vi "apply settings.vi"(8 "error in (no error)":errorcluster, 9 "selectors":T1, 10 "settings":string, 11 "refnum":refnum<vi>) -> (0 "error out":errorcluster)   [LabVIEW 2024, in "controls manager.lvlib"]
uses:
  controls manager.lvlib
  selectors.ctl
  <vilib>/Utility/error.llb/Trim Whitespace One-Sided.vi
  <vilib>/Utility/error.llb/Error Cluster From Error Code.vi
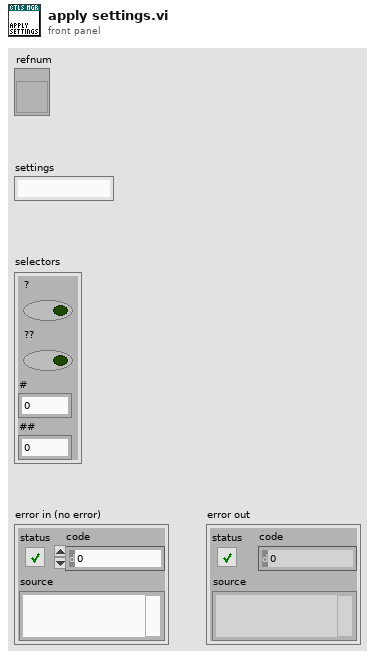
[diagram p1: front panel]
types:
  T1 = typedef "controls manager.lvlib/selectors.ctl" = cluster{"?":bool, "??":bool, "#":u16, "##":u16}
  T2 = enum8{"Enabled", "Disabled", "Disabled and Grayed Out"}
  T3 = typedef "controls manager.lvlib/keywords.ctl" = enum16{"___", "enable", "disable", "gray", "visible", "hidden", "tip", "caption", "blinking", "not_blinking", "page", "default"}
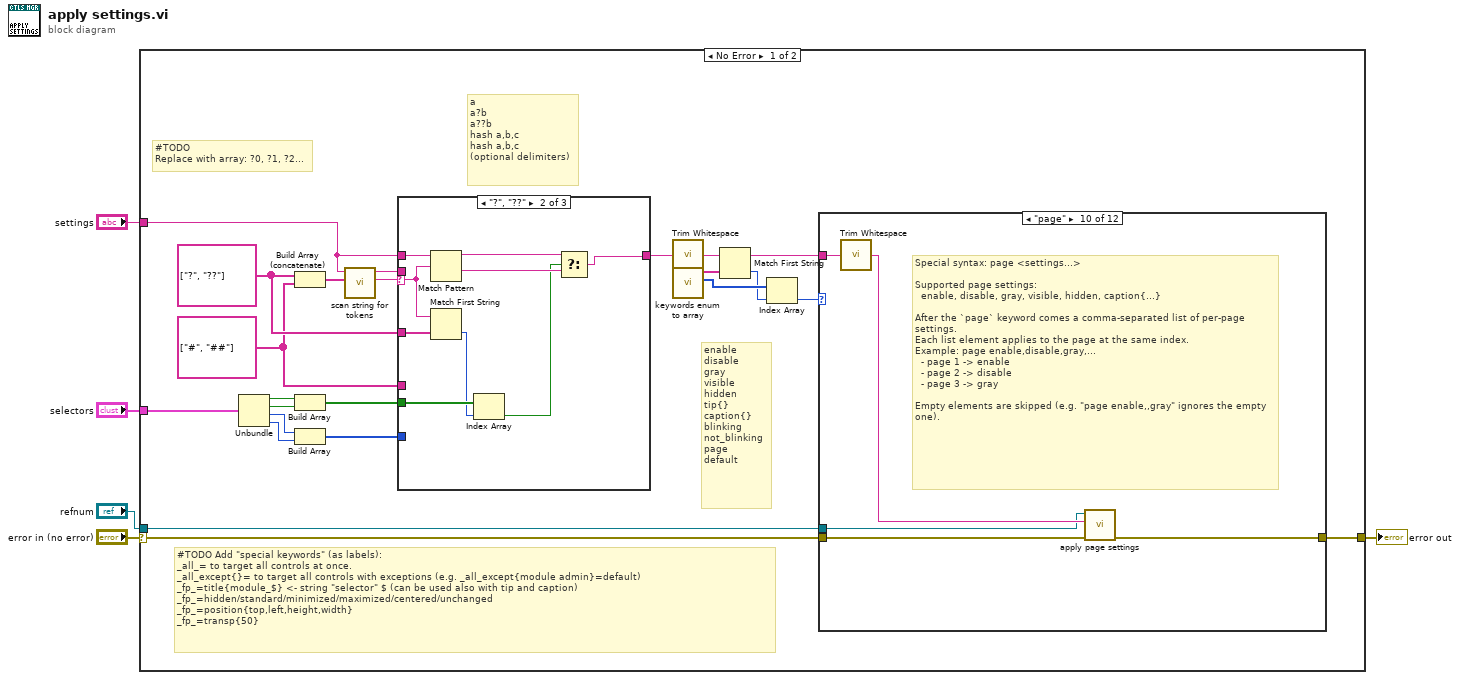
[diagram p0: block diagram]
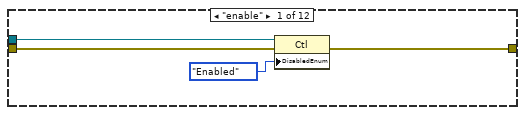
[diagram p2: hidden frame]
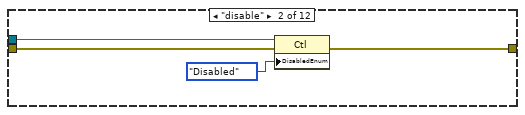
[diagram p3: hidden frame]
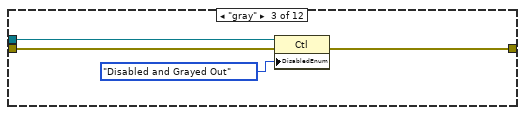
[diagram p4: hidden frame]
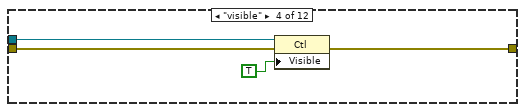
[diagram p5: hidden frame]
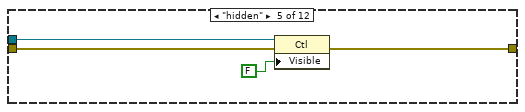
[diagram p6: hidden frame]
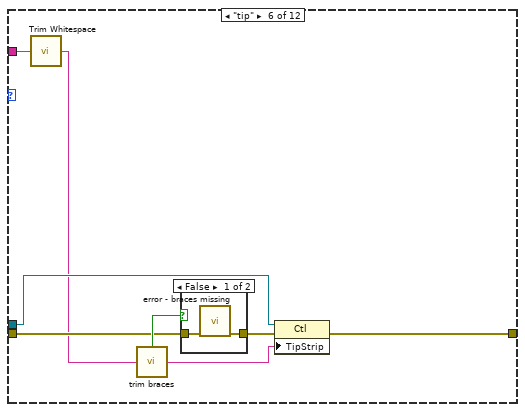
[diagram p7: hidden frame]
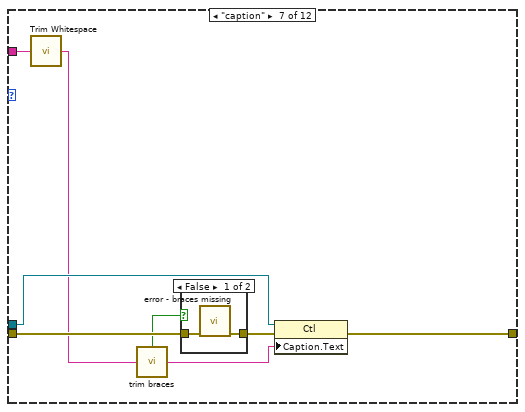
[diagram p9: hidden frame]
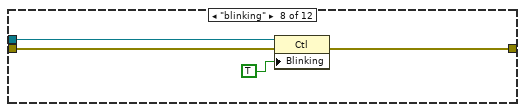
[diagram p11: hidden frame]
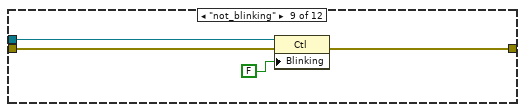
[diagram p12: hidden frame]
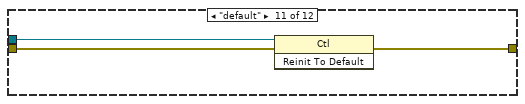
[diagram p13: hidden frame]
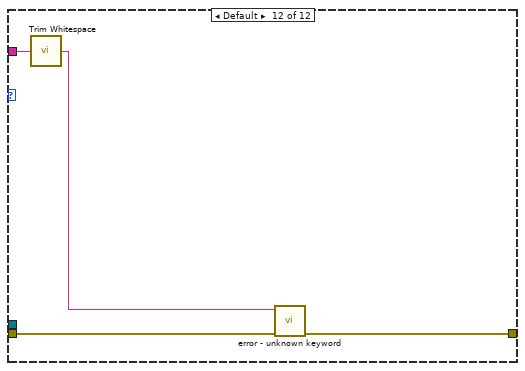
[diagram p14: hidden frame]
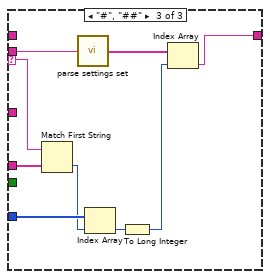
[diagram p16: hidden frame]
diagram:
  n1 = case shown="No Error" "error in (no error)" {
    selector: "error in (no error)" -> [w8 w110]
    tunnel: "settings" -> [w24 _]
    tunnel: "selectors" -> [w13 _]
    tunnel: [w7 w110] -> w2
    tunnel: "refnum" -> [w6 _]
    frame No Error {
      w14 = string[] ["#", "##"]
      w25 = string[] ["?", "??"]
      # "#TODO\nReplace with array: ?0, ?1, ?2..."
      # "#TODO Add \"special keywords\" (as labels):\n_all_= to target all controls at once.\n_all_except{}= to target all controls with exceptions (e.g. _all_except{module admin}=default)\n_fp_=title{module_$} <- string \"selector\" $ (can be used also with tip and caption)\n_fp_=hidden/standard/minimized/maximized/centered/unchanged\n_fp_=position{top,left,height,width}\n_fp_=transp{50}"
      # "enable\ndisable\ngray\nvisible\nhidden\ntip{}\ncaption{}\nblinking\nnot_blinking\npage\ndefault"
      # "a\na?b\na??b\nhash a,b,c\nhash a,b,c\n(optional delimiters)"
      n2 = Unbundle(w13) -> ("?"=w12:bool, "??"=w11:bool, "#"=w10:u16, "##"=w9:u16)
      n3 = Build Array (concatenate)(w25, w14) -> (w23:string[])
      n4 = Build Array(w12, w11) -> (w28:bool[])
      n5 = Build Array(w10, w9) -> (w27:u16[])
      n6 = call "scan string for tokens.vi"("operators"=w23, "input string"=w24) -> ("token string"=w22:string, "string out"=w21:string)  [unwired: 8 in]
      n7 = case shown="\"?\", \"??\"" w22 {
        selector: w22 -> [_ w98 w108]
        tunnel: w25 -> [_ w99 _]
        tunnel: w24 -> [w91 w97 _]
        tunnel: w28 -> [_ w96 _]
        tunnel: [w91 w92 w103] -> w16
        tunnel: w27 -> [_ _ w109]
        tunnel: w14 -> [_ _ w106]
        tunnel: w21 -> [_ _ w101]
        frame Default {
        }
        frame "?", "??" {
          n8 = Match Pattern(string=w97, regular expression=w98) -> (before substring=w93:string, after substring=w100:string)  [unwired: 1 in, 2 out]
          n9 = Match First String(2:w99, 3:w98) -> (0:w95:i32)  [unwired: 1 out]
          n10 = Index Array(array=w96, index=w95) -> (element=w94:bool)
          n11 = Select(t=w93, s=w94, f=w100) -> (s? t:f=w92:string)
        }
        frame "#", "##" {
          n12 = Match First String(2:w106, 3:w108) -> (0:w107:i32)  [unwired: 1 out]
          n13 = call "parse settings set.vi"("settings in"=w101) -> ("settings out"=w102:string[])
          n14 = Index Array(array=w109, index=w107) -> (element=w105:u16)
          n15 = To Long Integer(number=w105) -> (32bit integer=w104:i32)
          n16 = Index Array(array=w102, index=w104) -> (element=w103:string)
        }
      }
      n17 = call <vilib>:"Trim Whitespace.vi"("string"=w16) -> ("trimmed string"=w15:string)  [unwired: 1 in]
      n18 = call "keywords enum to array.vi"() -> ("enums"=w20:T3[], "strings"=w19:string[])  [unwired: 10 in]
      n19 = Match First String(2:w19, 3:w15) -> (0:w18:i32, 1:w17:string)
      n20 = Index Array(array=w20, index=w18) -> (element=w26:T3)
      n21 = case shown="\"page\"" w26 {
        tunnel: w17 -> [_ _ _ _ _ w55 w65 _ _ w81 _ w88]
        tunnel: w8 -> [w31 w35 w39 w44 w48 w53 w67 w74 w78 w83 w86 w90]
        tunnel: [w30 w34 w38 w43 w47 w56 w66 w73 w77 w82 w85 w89] -> w7
        tunnel: w6 -> [w29 w33 w37 w42 w46 w50 w61 w72 w76 w79 w84 _]
        frame "enable" {
          n22 = property class="Ctl"(reference=w29, error in=w31, "DisabledEnum"=T2."Enabled") -> (error out=w30:errorcluster)  [unwired: 1 out]
        }
        frame "disable" {
          n23 = property class="Ctl"(reference=w33, error in=w35, "DisabledEnum"=T2."Disabled") -> (error out=w34:errorcluster)  [unwired: 1 out]
        }
        frame "gray" {
          n24 = property class="Ctl"(reference=w37, error in=w39, "DisabledEnum"=T2."Disabled and Grayed Out") -> (error out=w38:errorcluster)  [unwired: 1 out]
        }
        frame "visible" {
          n25 = property class="Ctl"(reference=w42, error in=w44, "Visible"=TRUE) -> (error out=w43:errorcluster)  [unwired: 1 out]
        }
        frame "hidden" {
          n26 = property class="Ctl"(reference=w46, error in=w48, "Visible"=FALSE) -> (error out=w47:errorcluster)  [unwired: 1 out]
        }
        frame "tip" {
          n27 = call <vilib>:"Trim Whitespace.vi"("string"=w55) -> ("trimmed string"=w49:string)  [unwired: 1 in]
          n28 = call "trim braces.vi"("string"=w49) -> ("braces?"=w54:bool, "trimmed string"=w51:string)
          n29 = case shown="False" w54 {
            tunnel: w53 -> [w58 w59]
            tunnel: [w57 w59] -> w52
            frame False {
              n30 = call "error - braces missing.vi"("error in (no error)"=w58) -> ("error out"=w57:errorcluster)  [unwired: 10 in]
            }
            frame True {
            }
          }
          n31 = property class="Ctl"(reference=w50, error in=w52, "TipStrip"=w51) -> (error out=w56:errorcluster)  [unwired: 1 out]
        }
        frame "caption" {
          n32 = call <vilib>:"Trim Whitespace.vi"("string"=w65) -> ("trimmed string"=w60:string)  [unwired: 1 in]
          n33 = call "trim braces.vi"("string"=w60) -> ("braces?"=w64:bool, "trimmed string"=w62:string)
          n34 = case shown="False" w64 {
            tunnel: w67 -> [w69 w70]
            tunnel: [w68 w70] -> w63
            frame False {
              n35 = call "error - braces missing.vi"("error in (no error)"=w69) -> ("error out"=w68:errorcluster)  [unwired: 10 in]
            }
            frame True {
            }
          }
          n36 = property class="Ctl"(reference=w61, error in=w63, "Caption.Text"=w62) -> (error out=w66:errorcluster)  [unwired: 1 out]
        }
        frame "blinking" {
          n37 = property class="Ctl"(reference=w72, error in=w74, "Blinking"=TRUE) -> (error out=w73:errorcluster)  [unwired: 1 out]
        }
        frame "not_blinking" {
          n38 = property class="Ctl"(reference=w76, error in=w78, "Blinking"=FALSE) -> (error out=w77:errorcluster)  [unwired: 1 out]
        }
        frame "page" {
          # "Special syntax: page <settings...>\n\nSupported page settings:\n  enable, disable, gray, visible, hidden, caption{...}\n\nAfter the `page` keyword comes a comma-separated list of per-page settings.\nEach list element applies to the page at the same index.\nExample: page enable,disable,gray,...\n  - page 1 -> enable\n  - page 2 -> disable\n  - page 3 -> gray\n\nEmpty elements are skipped (e.g. \"page enable,,gray\" ignores the empty one)."
          n39 = call <vilib>:"Trim Whitespace.vi"("string"=w81) -> ("trimmed string"=w80:string)  [unwired: 1 in]
          n40 = call "apply page settings.vi"("error in (no error)"=w83, "page settings"=w80, "tab control refnum"=w79) -> ("error out"=w82:errorcluster)  [unwired: 8 in]
        }
        frame "default" {
          n41 = invoke class="Ctl" method="Reinit To Default"(reference=w84, error in=w86) -> (error out=w85:errorcluster)  [unwired: 1 in, 2 out]
        }
        frame Default {
          n42 = call <vilib>:"Trim Whitespace.vi"("string"=w88) -> ("trimmed string"=w87:string)  [unwired: 1 in]
          n43 = call "error - unknown keyword.vi"("error in (no error)"=w90, "keyword"=w87) -> ("error out"=w89:errorcluster)  [unwired: 9 in]
        }
      }
    }
    frame Error {
    }
  }
  "error out" <- w2
